vi "draw_feature_subVI.vi"(6 "Color":u32(colorbox)=65280, 8 "Error In":errorcluster, 10 "Feature Ponts":cluster{"X":sgl, "Y":sgl}[](array[cluster]), 11 "Image":T1) -> (0 "Error Out":errorcluster, 3 "Image Out":T1)   [LabVIEW 2014]
uses:
  <vilib>/vision/Image Controls.llb/IMAQ Image.ctl
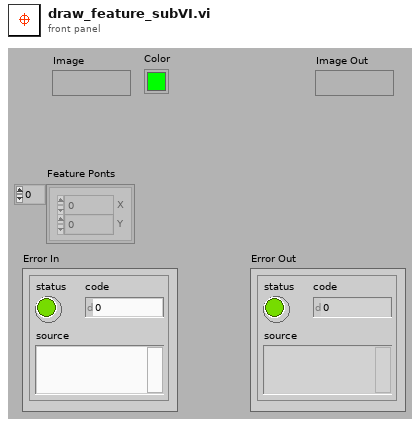
[diagram p1: front panel]
types:
  T1 = typedef "IMAQ Image.ctl" = refnum<image>
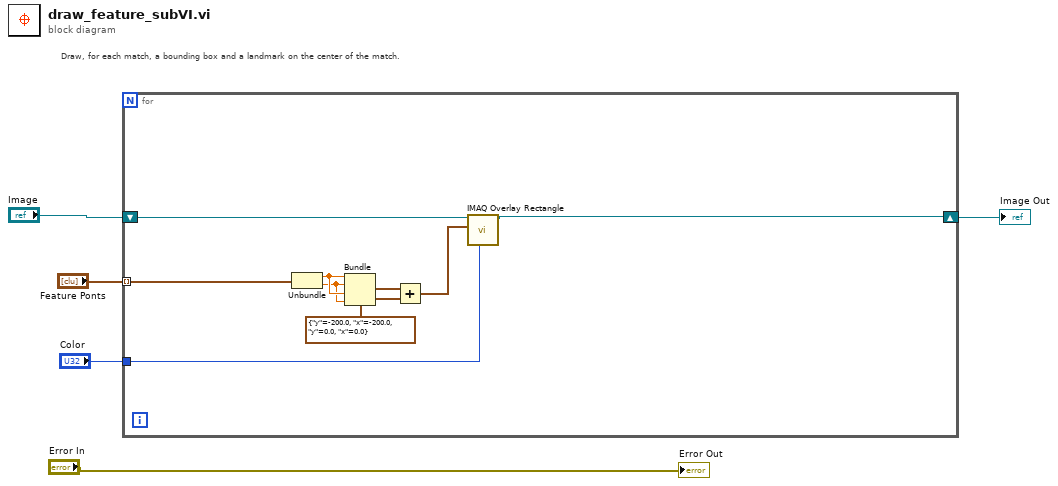
[diagram p0: block diagram]
diagram:
  # "Draw, for each match, a bounding box and a landmark on the center of the match."
  n1 = for {
    shift-right: [w6] -> w4
    shift-left: "Image" -> [w14]
    tunnel: "Feature Ponts" -> [w12] mode=indexing
    tunnel: "Color" -> [w13]
    n2 = Unbundle(w12) -> ("X"=w11:sgl, "Y"=w10:sgl)
    n3 = Bundle("X"=w11, "Y"=w10, "X"=w11, "Y"=w10) -> (w9:cluster{"X":sgl, "Y":sgl, "X":sgl, "Y":sgl})  [unwired: 1 out]
    n4 = Add(x=w9, y=cluster{"y":sgl, "x":sgl, "y":sgl, "x":sgl} {"y"=-200.0, "x"=-200.0, "y"=0.0, "x"=0.0}) -> (x+y=w7:cluster{sgl, sgl, sgl, sgl})
    n5 = call "IMAQ Overlay Rectangle"("Color"=w13, "Rectangle"=w7, "Image"=w14) -> ("Image Out"=w6:T1)  [unwired: 7 in, 1 out]
  }
  "Image Out" <- w4
  "Error Out" <- "Error In"
